vi "CallbackExample - MAIN.vi"() -> ()   [LabVIEW 2011]
doc: "Demonstration VI that calls the call back VI and demonstrates how one call back can change functionality in a way that is similar to a drop in.\n\nAAL 9/09"
panel:
  in  "Tree 3":string(tree)="SubItem1"
  in  "Tree 2":string(tree)="Item 2"
  in  "stop":bool
  in  "Tree":string(tree)
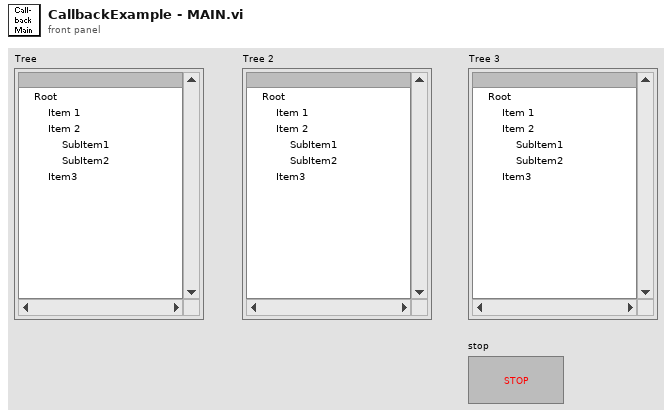
[diagram p1: front panel]
types:
  T1 = cluster{"Unchecked Item":i32, "Checked Item":i32}
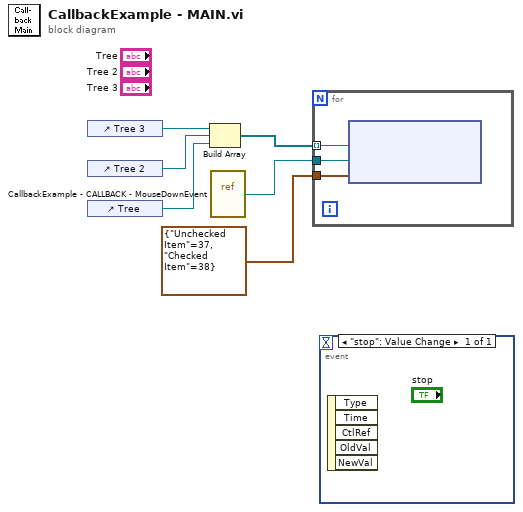
[diagram p0: block diagram]
diagram:
  n1 = control-ref of="Tree 3"() -> (w1:refnum<vi>)
  n2 = control-ref of="Tree 2"() -> (w3:refnum<vi>)
  n3 = control-ref of="Tree"() -> (w2:refnum<vi>)
  n4 = Build Array(w1, w3, w2) -> (w4:refnum<vi>[])
  n5 = vi-ref "CallbackExample - CALLBACK - MouseDownEvent.vi"() -> ("vi reference"=w5:refnum<vi>)
  n6 = for {
    tunnel: T1 {"Unchecked Item"=37, "Checked Item"=38} ("Cluster") -> [w9]
    tunnel: w5 -> [w8]
    tunnel: w4 -> [w7] mode=indexing
    n7 = node(w7, w8, w9) -> ()  [unwired: 2 in, 2 out]
  }
  n8 = event shown="[0] \"stop\": Value Change" {
    selector: _ -> [_]
    dyn-events: _ -> [_]
    timeout: _ -> [_]
    event "stop": Value Change {
      n9 = event-data() -> ()  [unwired: 1 in, 5 out]
    }
  }
